vi "Create Clip Planes.vi"(8 "error in (no error)":errorcluster, 10 "Terrain Size":dbl, 11 "Main Scene Object Ref":refnum<vi>) -> (0 "error out":errorcluster, 3 "Main Scene Object Ref (out)":refnum<vi>)   [LabVIEW 2023]
uses:
  <vilib>/picture/3D Picture Control/Helpers/Set Clip Plane (no reference).vi
  <vilib>/picture/3D Picture Control/NI_3D Picture Control.lvlib
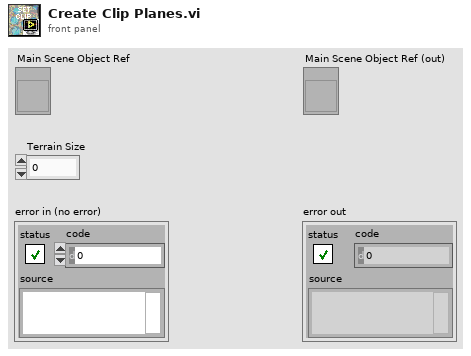
[diagram p1: front panel]
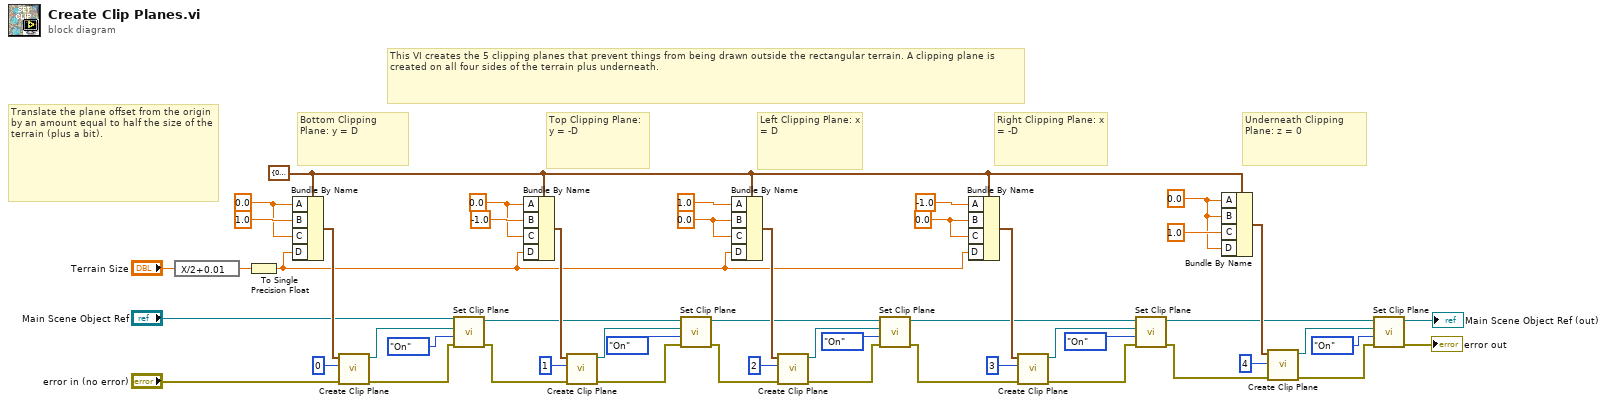
[diagram p0: block diagram]
diagram:
  w33 = sgl 0.0 ("A")
  w37 = sgl 0.0 ("B")
  w38 = sgl 0.0 ("B")
  w47 = sgl 0.0 ("A")
  w49 = sgl 0.0 ("A")
  w32 = cluster{"A":sgl, "B":sgl, "C":sgl, "D":sgl} {"A"=0.0, "B"=0.0, "C"=0.0, "D"=0.0} ("Plane")
  # "This VI creates the 5 clipping planes that prevent things from being drawn outside the rectangular terrain. A clipping plane is created on all four sides of the terrain plus underneath."
  # "Translate the plane offset from the origin by an amount equal to half the size of the terrain (plus a bit)."
  # "Underneath Clipping Plane: z = 0"
  # "Right Clipping Plane: x = -D"
  # "Left Clipping Plane: x = D"
  # "Top Clipping Plane: y = -D"
  # "Bottom Clipping Plane: y = D"
  n1 = expression code="X/2+0.01"("Terrain Size") -> (w2:dbl)
  n2 = To Single Precision Float(number=w2) -> (single precision float=w3:sgl)
  n3 = Bundle By Name(cluster=w32, "A"=w49, "B"=sgl 1.0, "C"=w49, "D"=w3) -> (w46:cluster{"A":sgl, "B":sgl, "C":sgl, "D":sgl})
  n4 = call <vilib>:"Create Clip Plane.vi"("error in (no error)"="error in (no error)", "Number"=0, "Plane"=w46) -> ("error out"=w28:errorcluster, "New Clip Plane Refnum"=w26:refnum<vi>)  [unwired: 7 out]
  n5 = call-poly <vilib>:"Set Clip Plane.vi"("error in (no error)"=w28, "Clip Plane State"=enum16{"Inherit Value", "Off", "On"}."On", "Clip Plane Refnum In"=w26, "Scene Object In"="Main Scene Object Ref") -> ("error out"=w4:errorcluster, "Scene Object Out"=w25:refnum<vi>)  [unwired: 6 in]
  n6 = Bundle By Name(cluster=w32, "A"=w47, "B"=sgl -1.0, "C"=w47, "D"=w3) -> (w45:cluster{"A":sgl, "B":sgl, "C":sgl, "D":sgl})
  n7 = call <vilib>:"Create Clip Plane.vi"("error in (no error)"=w4, "Number"=1, "Plane"=w45) -> ("error out"=w5:errorcluster, "New Clip Plane Refnum"=w24:refnum<vi>)  [unwired: 7 out]
  n8 = call-poly <vilib>:"Set Clip Plane.vi"("error in (no error)"=w5, "Clip Plane State"=enum16{"Inherit Value", "Off", "On"}."On", "Clip Plane Refnum In"=w24, "Scene Object In"=w25) -> ("error out"=w6:errorcluster, "Scene Object Out"=w22:refnum<vi>)  [unwired: 6 in]
  n9 = Bundle By Name(cluster=w32, "A"=sgl 1.0, "B"=w38, "C"=w38, "D"=w3) -> (w41:cluster{"A":sgl, "B":sgl, "C":sgl, "D":sgl})
  n10 = call <vilib>:"Create Clip Plane.vi"("error in (no error)"=w6, "Number"=2, "Plane"=w41) -> ("error out"=w7:errorcluster, "New Clip Plane Refnum"=w21:refnum<vi>)  [unwired: 7 out]
  n11 = call-poly <vilib>:"Set Clip Plane.vi"("error in (no error)"=w7, "Clip Plane State"=enum16{"Inherit Value", "Off", "On"}."On", "Clip Plane Refnum In"=w21, "Scene Object In"=w22) -> ("error out"=w8:errorcluster, "Scene Object Out"=w18:refnum<vi>)  [unwired: 6 in]
  n12 = Bundle By Name(cluster=w32, "A"=sgl -1.0, "B"=w37, "C"=w37, "D"=w3) -> (w36:cluster{"A":sgl, "B":sgl, "C":sgl, "D":sgl})
  n13 = call <vilib>:"Create Clip Plane.vi"("error in (no error)"=w8, "Number"=3, "Plane"=w36) -> ("error out"=w9:errorcluster, "New Clip Plane Refnum"=w17:refnum<vi>)  [unwired: 7 out]
  n14 = call-poly <vilib>:"Set Clip Plane.vi"("error in (no error)"=w9, "Clip Plane State"=enum16{"Inherit Value", "Off", "On"}."On", "Clip Plane Refnum In"=w17, "Scene Object In"=w18) -> ("error out"=w10:errorcluster, "Scene Object Out"=w16:refnum<vi>)  [unwired: 6 in]
  n15 = Bundle By Name(cluster=w32, "A"=w33, "B"=w33, "C"=sgl 1.0 ("B"), "D"=w33) -> (w31:cluster{"A":sgl, "B":sgl, "C":sgl, "D":sgl})
  n16 = call <vilib>:"Create Clip Plane.vi"("error in (no error)"=w10, "Number"=4, "Plane"=w31) -> ("error out"=w11:errorcluster, "New Clip Plane Refnum"=w15:refnum<vi>)  [unwired: 7 out]
  n17 = call-poly <vilib>:"Set Clip Plane.vi"("error in (no error)"=w11, "Clip Plane State"=enum16{"Inherit Value", "Off", "On"}."On", "Clip Plane Refnum In"=w15, "Scene Object In"=w16) -> ("error out"=→"error out":errorcluster, "Scene Object Out"=→"Main Scene Object Ref (out)":refnum<vi>)  [unwired: 6 in]
